vi "stop listening.vi"(8 "error in":errorcluster, 11 "TCP server in":refnum<class "TCP server.lvclass">) -> (0 "error out":errorcluster, 3 "TCP server out":refnum<class "TCP server.lvclass">)   [LabVIEW 2015, in "TCP server.lvclass"]
uses:
  TCP server.lvclass
  TCP server.lvclass/TCP server.ctl
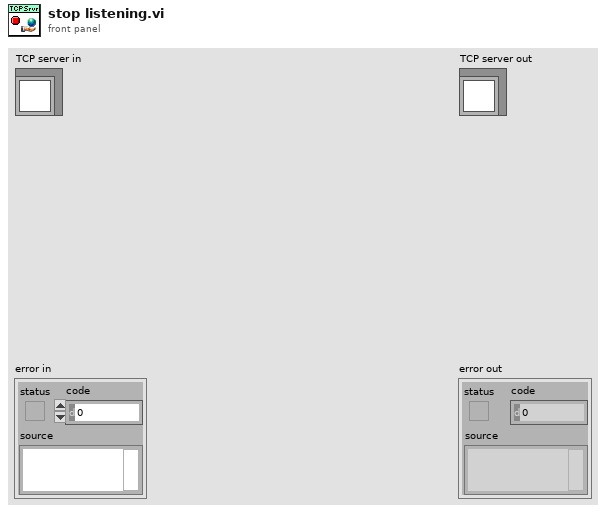
[diagram p1: front panel]
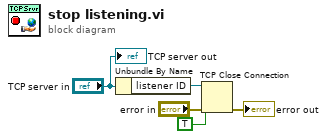
[diagram p0: block diagram]
diagram:
  n1 = Unbundle By Name("TCP server in") -> ("listener ID"=w2:refnum<k5>)
  n2 = TCP Close Connection(connection ID=w2, abort (F)=TRUE, error in (no error)="error in") -> (error out=→"error out":errorcluster)  [unwired: 1 out]
  "TCP server out" <- "TCP server in"
